vi "MapItemNametoSymbol.vi"(4 "Item Name":string) -> (1 "Symbol Index":i32)   [LabVIEW 2010]
doc: "Creates mapping between item names (tags) and custom symbol index."
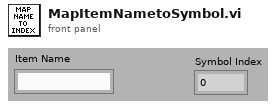
[diagram p1: front panel]
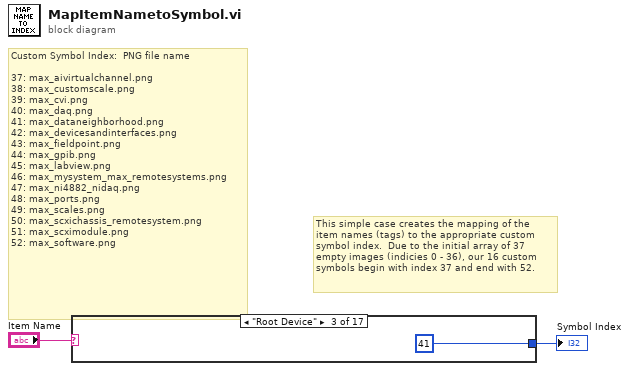
[diagram p0: block diagram]
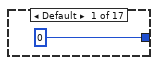
[diagram p2: hidden frame]
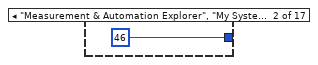
[diagram p3: hidden frame]
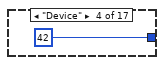
[diagram p4: hidden frame]
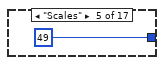
[diagram p5: hidden frame]
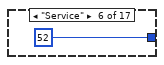
[diagram p6: hidden frame]
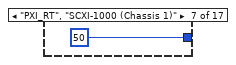
[diagram p7: hidden frame]
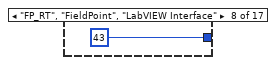
[diagram p8: hidden frame]
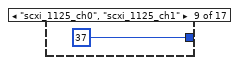
[diagram p9: hidden frame]
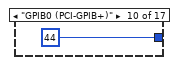
[diagram p10: hidden frame]
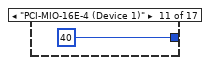
[diagram p11: hidden frame]
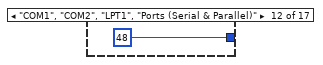
[diagram p12: hidden frame]
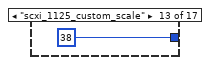
[diagram p13: hidden frame]
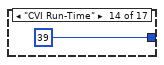
[diagram p14: hidden frame]
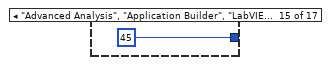
[diagram p15: hidden frame]
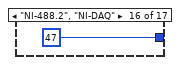
[diagram p16: hidden frame]
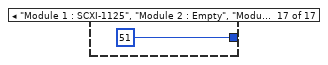
[diagram p17: hidden frame]
diagram:
  # "This simple case creates the mapping of the\nitem names (tags) to the appropriate custom\nsymbol index.  Due to the initial array of 37\nempty images (indicies 0 - 36), our 16 custom\nsymbols begin with index 37 and end with 52."
  # "Custom Symbol Index:  PNG file name\n\n37: max_aivirtualchannel.png\n38: max_customscale.png\n39: max_cvi.png\n40: max_daq.png\n41: max_dataneighborhood.png\n42: max_devicesandinterfaces.png\n43: max_fieldpoint.png\n44: max_gpib.png\n45: max_labview.png\n46: max_mysystem_max_remotesystems.png\n47: max_ni4882_nidaq.png\n48: max_ports.png\n49: max_scales.png\n50: max_scxichassis_remotesystem.png\n51: max_scximodule.png\n52: max_software.png"
  n1 = case shown="\"Root Device\"" "Item Name" {
    tunnel: [0 46 41 42 49 52 50 43 37 44 40 48 38 39 45 47 51] -> w1
    frame Default {
    }
    frame "Measurement & Automation Explorer", "My System", "Remote Systems" {
    }
    frame "Root Device" {
    }
    frame "Device" {
    }
    frame "Scales" {
    }
    frame "Service" {
    }
    frame "PXI_RT", "SCXI-1000 (Chassis 1)" {
    }
    frame "FP_RT", "FieldPoint", "LabVIEW Interface" {
    }
    frame "scxi_1125_ch0", "scxi_1125_ch1" {
    }
    frame "GPIB0 (PCI-GPIB+)" {
    }
    frame "PCI-MIO-16E-4 (Device 1)" {
    }
    frame "COM1", "COM2", "LPT1", "Ports (Serial & Parallel)" {
    }
    frame "scxi_1125_custom_scale" {
    }
    frame "CVI Run-Time" {
    }
    frame "Advanced Analysis", "Application Builder", "LabVIEW", "LabVIEW Run-Time" {
    }
    frame "NI-488.2", "NI-DAQ" {
    }
    frame "Module 1 : SCXI-1125", "Module 2 : Empty", "Module 3 : Empty", "Module 4 : Empty" {
    }
  }
  "Symbol Index" <- w1
